vi "Command Lifter to Setpoint.vi"(2 "Input Robot System Funtions":T1, 3 "Cmd Parameter 1":dbl, 4 "Cmd Parameter 2":dbl, 5 "Startup":bool) -> (0 "Output Robot System Functions":T1, 1 "Completed":bool)   [LabVIEW 2014]
uses:
  Subsystems VIs/Robot Commands.ctl
  Command Execution State.ctl
  Global Variables/Miscalleneous.vi
  Global Variables/Sensor Data (Edited).vi
panel:
  # "Sample robot\ncontrol output.\nReplace with \nactual teleop \ncontrol signal \nstructure."
  # "Field Centric"
  # "Field Centric"
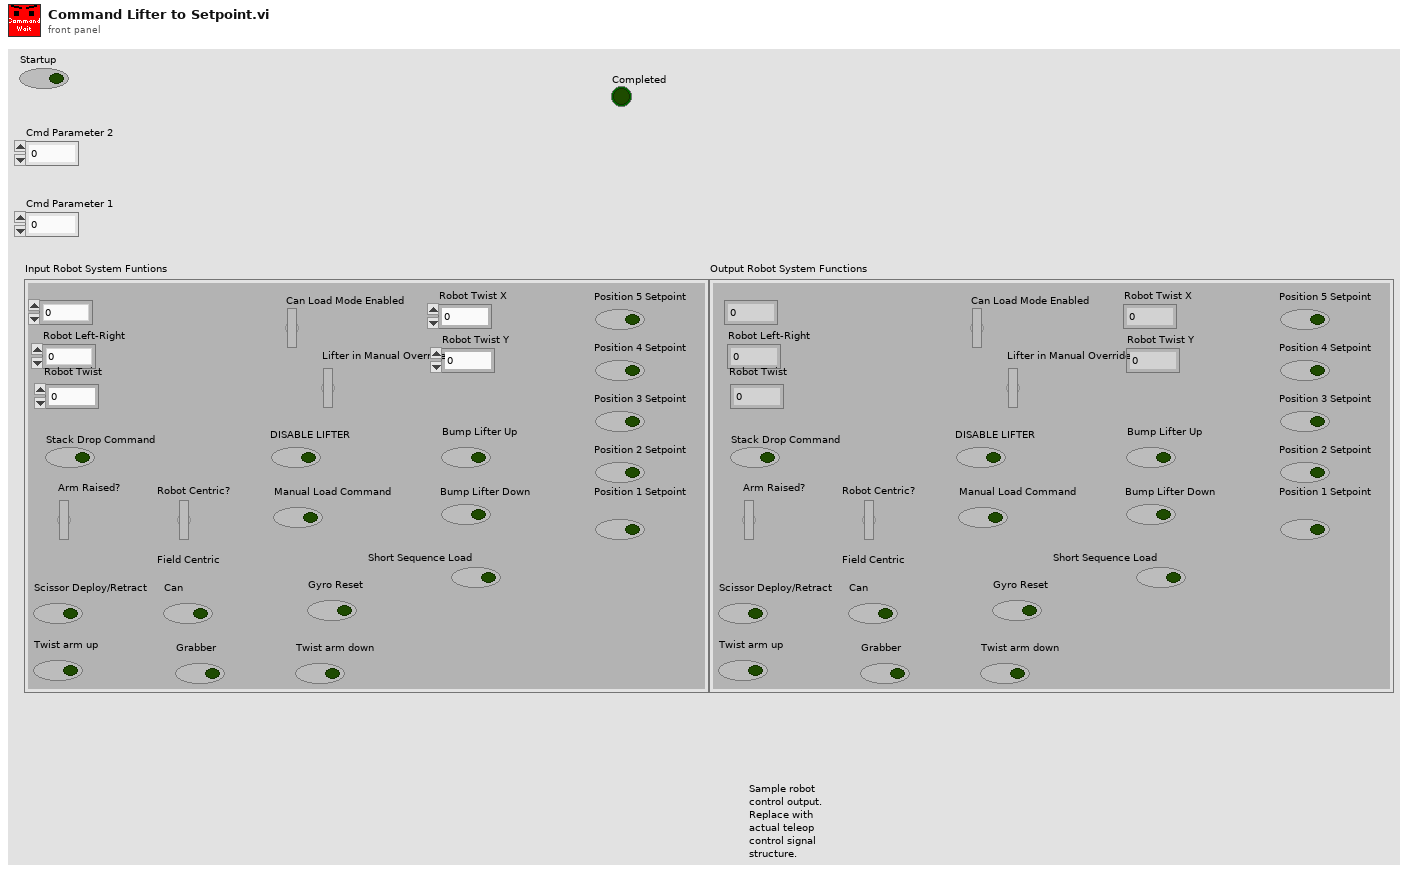
[diagram p1: front panel]
types:
  T1 = typedef "Robot Commands.ctl" = cluster{"Robot Forward-Reverse":dbl, "Robot Left-Right":dbl, "Robot Twist":dbl, "Can Load Mode Enabled":bool, "Lifter in Manual Override?":bool, "Stack Drop Command":bool, "Arm Raised?":bool, "DISABLE LIFTER":bool, "Position 1 Setpoint":bool, "Position 2 Setpoint":bool, "Position 3 Setpoint":bool, "Position 4 Setpoint":bool, "Position 5 Setpoint":bool, "Bump Lifter Down":bool, "Bump Lifter Up":bool, "Manual Load Command":bool, "Robot Centric?":bool, "Scissor Deploy/Retract":bool, "Grabber":bool, "Can":bool, "Twist arm up":bool, "Gyro Reset":bool, "Twist arm down":bool, "Short Sequence Load":bool, "Robot Twist X":dbl, "Robot Twist Y":dbl}
  T2 = typedef "Command Execution State.ctl" = enum16{"Initialize", "Execute", "Finish"}
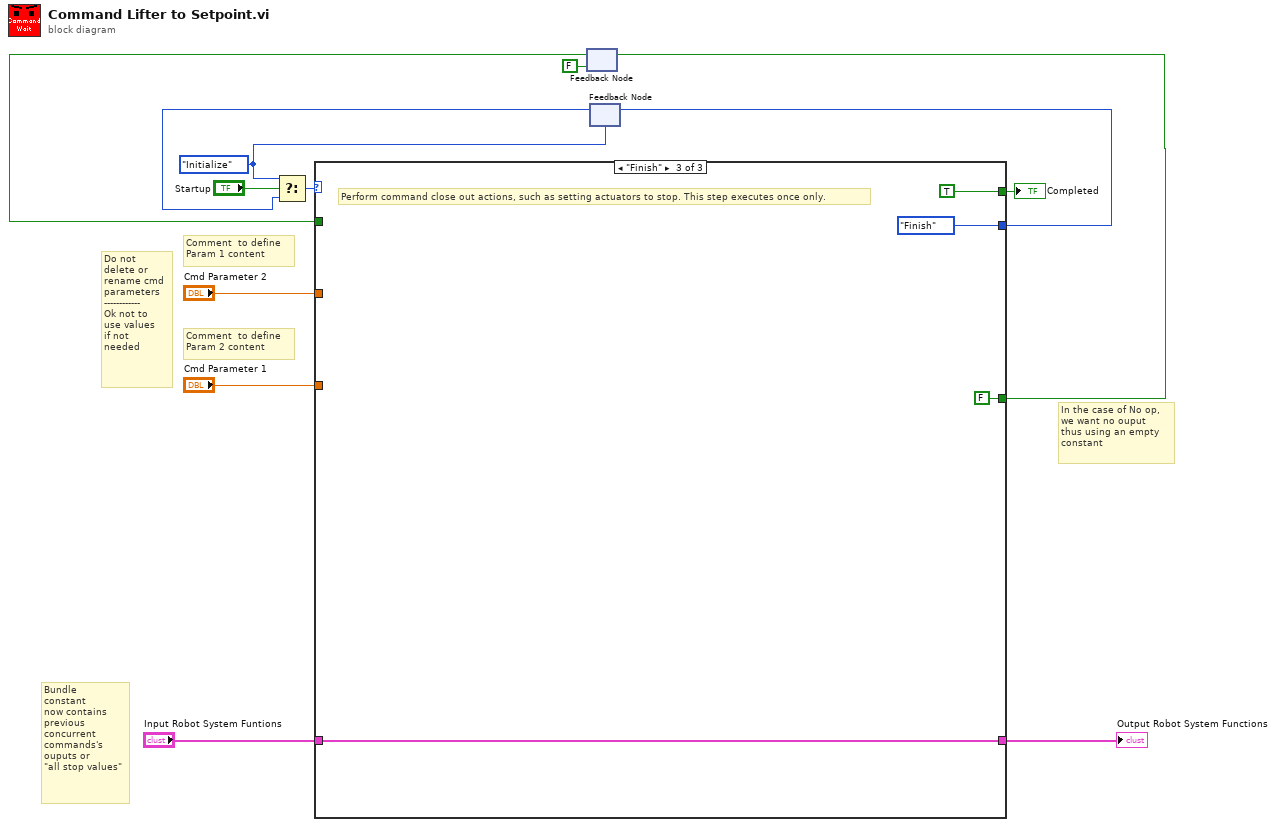
[diagram p0: block diagram]
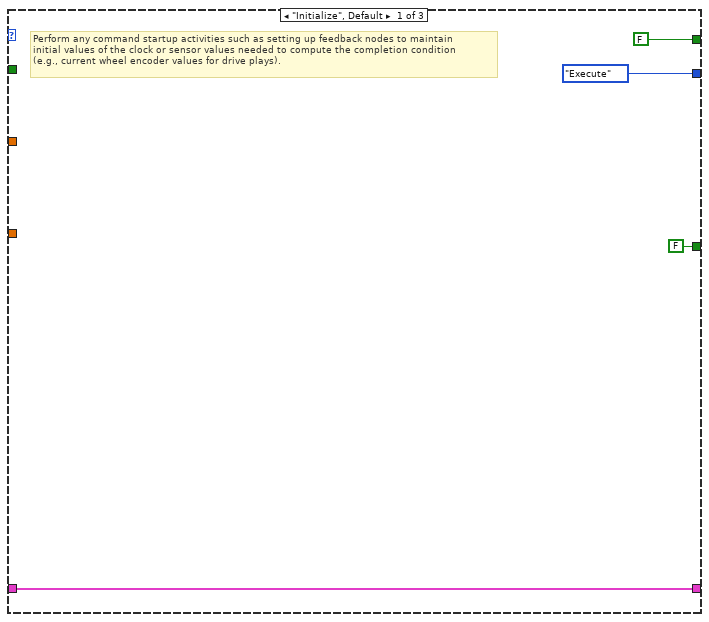
[diagram p2: hidden frame]
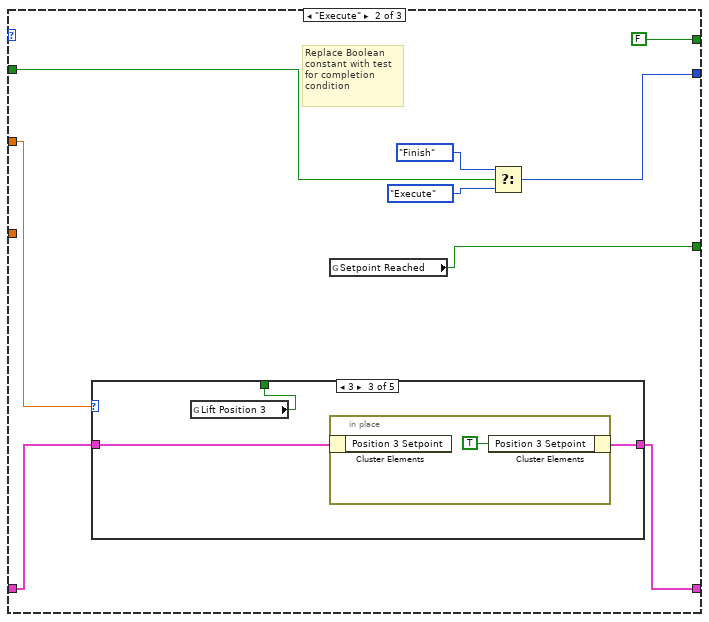
[diagram p3: hidden frame]
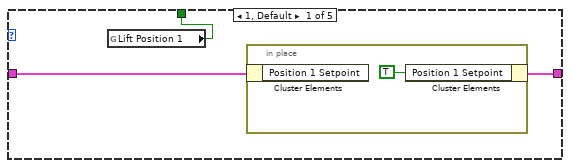
[diagram p4: hidden frame]
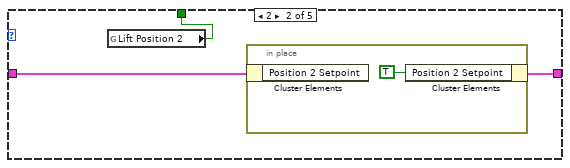
[diagram p5: hidden frame]
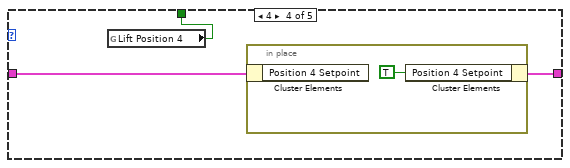
[diagram p6: hidden frame]
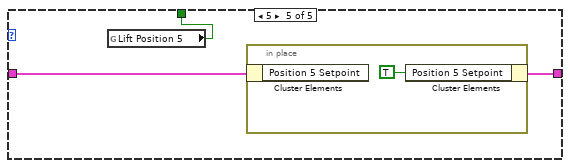
[diagram p7: hidden frame]
diagram:
  w8 = Command_Execution_State."Initialize" ("Play State")
  # "In the case of No op, \nwe want no ouput \nthus using an empty \nconstant"
  # "Bundle \nconstant\nnow contains\nprevious \nconcurrent\ncommands's\nouputs or\n\"all stop values\""
  # "Do not \ndelete or\nrename cmd\nparameters\n------------\nOk not to \nuse values\nif not \nneeded"
  # "Comment  to define\nParam 2 content"
  # "Comment  to define\nParam 1 content"
  n1 = feedback #1(FALSE ("Setpoint Reached")) -> (w2:bool)
  n2 = feedback #2(w8) -> (w9:T2)
  n3 = Select(t=w8, s="Startup", f=w9) -> (s? t:f=w13:T2)
  n4 = case shown="\"Finish\"" w13 {
    tunnel: [FALSE FALSE TRUE] -> w11
    tunnel: [Command_Execution_State."Execute" ("Play State") w20 Command_Execution_State."Finish" ("f")] -> w10
    tunnel: "Cmd Parameter 2" -> [_ w23 _]
    tunnel: "Cmd Parameter 1" -> [_ _ _]
    tunnel: [w15 w24 w47] -> w4
    tunnel: "Input Robot System Funtions" -> [w15 w25 w47]
    tunnel: [FALSE ("Setpoint Reached") w19 FALSE ("Setpoint Reached")] -> w3
    tunnel: w2 -> [_ w18 _]
    frame "Initialize", Default {
      # "Perform any command startup activities such as setting up feedback nodes to maintain \ninitial values of the clock or sensor values needed to compute the completion condition\n(e.g., current wheel encoder values for drive plays)."
    }
    frame "Execute" {
      # "Replace Boolean\nconstant with test \nfor completion \ncondition"
      n5 = case shown="3" w23 {
        tunnel: w25 -> [w29 w33 w37 w41 w45]
        tunnel: [w28 w32 w36 w40 w44] -> w24
        tunnel: [w27 w31 w35 w39 w43] -> _
        frame 1, Default {
          n6 = global read "Sensor Data (Edited).vi" "Lift Position 1"() -> (w27:bool)
          n7 = in-place {
            n8 = in-place-cluster #3(w29) -> ()  [unwired: 1 out]
            n9 = in-place-cluster #3("Position 1 Setpoint"=TRUE) -> (w28:T1)
          }
        }
        frame 2 {
          n10 = global read "Sensor Data (Edited).vi" "Lift Position 2"() -> (w31:bool)
          n11 = in-place {
            n12 = in-place-cluster #4(w33) -> ()  [unwired: 1 out]
            n13 = in-place-cluster #4("Position 2 Setpoint"=TRUE ("Position 1 Setpoint")) -> (w32:T1)
          }
        }
        frame 3 {
          n14 = global read "Sensor Data (Edited).vi" "Lift Position 3"() -> (w35:bool)
          n15 = in-place {
            n16 = in-place-cluster #5(w37) -> ()  [unwired: 1 out]
            n17 = in-place-cluster #5("Position 3 Setpoint"=TRUE ("Position 1 Setpoint")) -> (w36:T1)
          }
        }
        frame 4 {
          n18 = global read "Sensor Data (Edited).vi" "Lift Position 4"() -> (w39:bool)
          n19 = in-place {
            n20 = in-place-cluster #6(w41) -> ()  [unwired: 1 out]
            n21 = in-place-cluster #6("Position 4 Setpoint"=TRUE ("Position 1 Setpoint")) -> (w40:T1)
          }
        }
        frame 5 {
          n22 = global read "Sensor Data (Edited).vi" "Lift Position 5"() -> (w43:bool)
          n23 = in-place {
            n24 = in-place-cluster #7(w45) -> ()  [unwired: 1 out]
            n25 = in-place-cluster #7("Position 5 Setpoint"=TRUE ("Position 1 Setpoint")) -> (w44:T1)
          }
        }
      }
      n26 = global read "Miscalleneous.vi" "Setpoint Reached"() -> (w19:bool)
      n27 = Select(t=Command_Execution_State."Finish" ("Play State"), s=w18, f=Command_Execution_State."Execute" ("Play State")) -> (s? t:f=w20:T2)
    }
    frame "Finish" {
      # "Perform command close out actions, such as setting actuators to stop. This step executes once only."
    }
  }
  "Completed" <- w11
  "Output Robot System Functions" <- w4
  n28 = feedback-in #1(w3) -> ()
  n29 = feedback-in #2(w10) -> ()
